vi "Configure Parameter to Measure.vi"(8 "error in (no error)":errorcluster, 10 "Sparameters (string)":string[](array[string]), 11 "VNA-PNA in":refnum<class "VNA-PNA.lvclass">) -> (0 "error out":errorcluster, 3 "VNA-PNA out":refnum<class "VNA-PNA.lvclass">)   [LabVIEW 2020, in "VNA-PNA.lvclass"]
doc: "Configures the active trace.\nIt creates the trace and sets the S paramert and mode."
uses:
  VNA-PNA.lvclass
  C:/Sandbox/RF Bench/Source Code/WiSpry Test Framework/Instruments/Vector Network Analyzer/Vector Network Analyzer.lvclass
  C:/Sandbox/RF Bench/Source Code/WiSpry Test Framework/Instruments/Instrument.lvclass
  Vector Network Analyzer.lvclass/Vector Network Analyzer.ctl
  Instrument.lvclass/Instrument.ctl
  Vector Network Analyzer.lvclass
  Instrument.lvclass
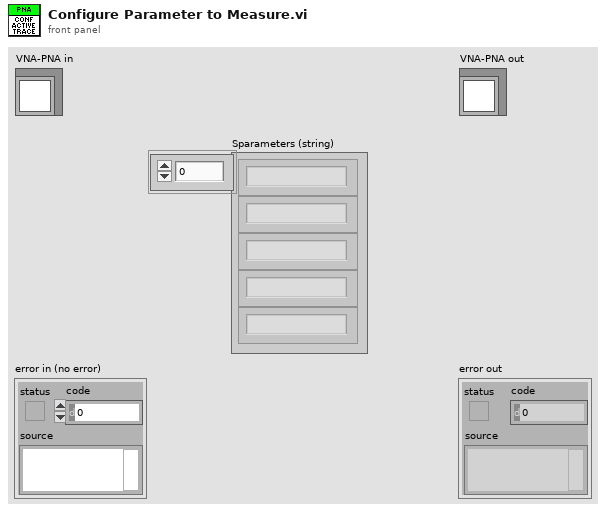
[diagram p1: front panel]
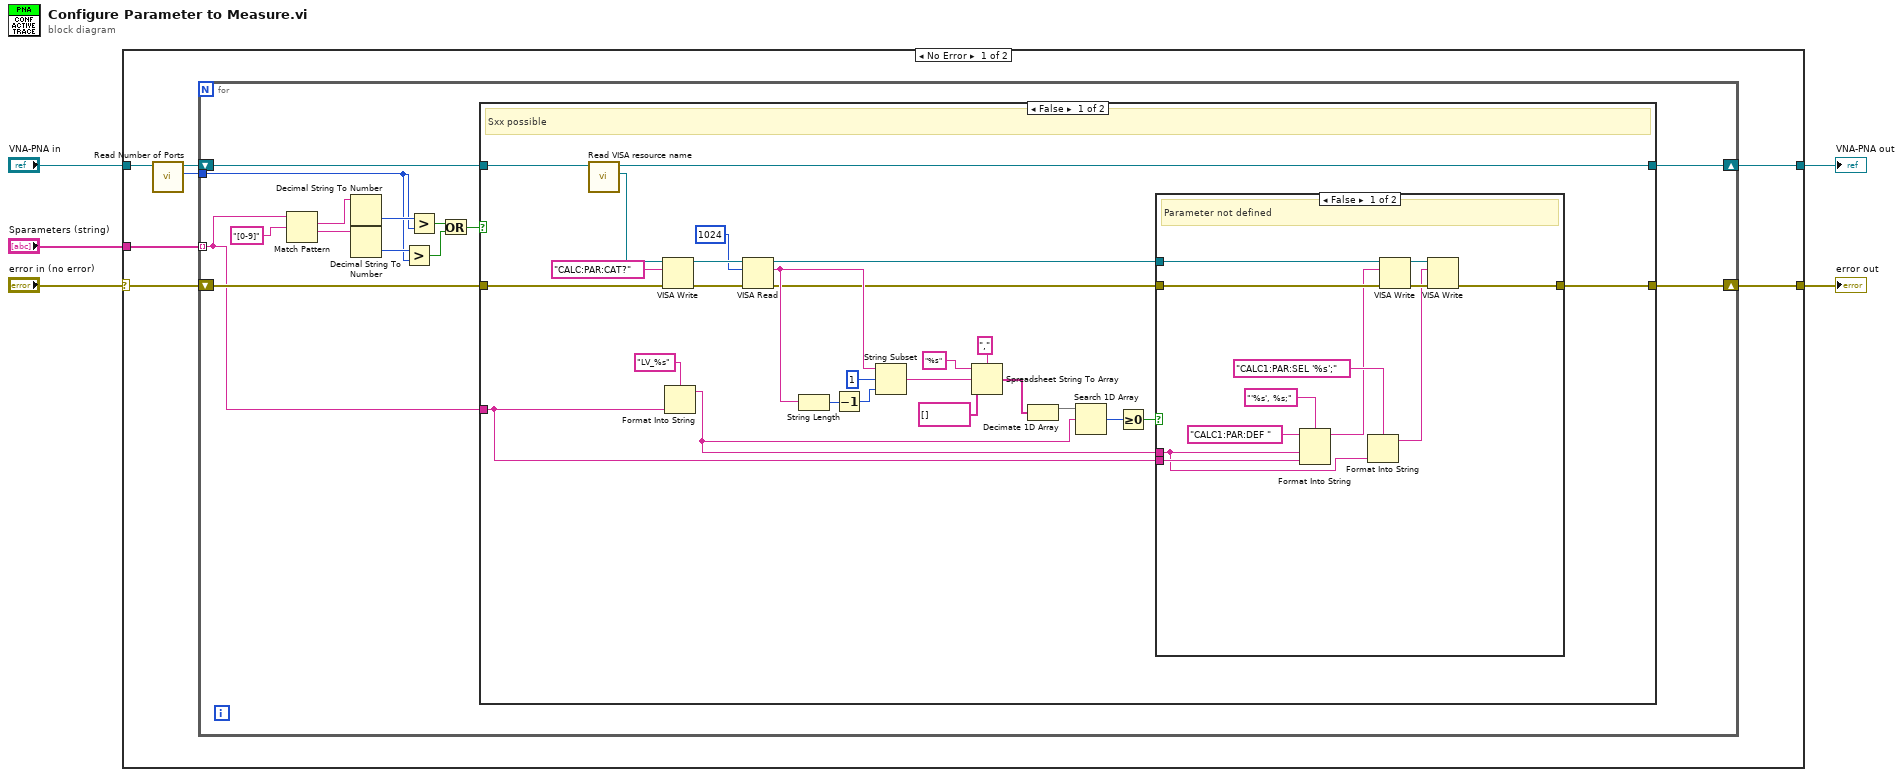
[diagram p0: block diagram]
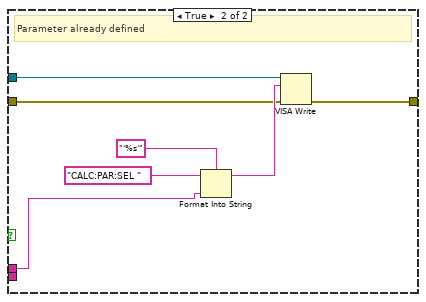
[diagram p2: hidden frame]
diagram:
  n1 = case shown="No Error" "error in (no error)" {
    selector: "error in (no error)" -> [w9 w75]
    tunnel: "VNA-PNA in" -> [w12 w74]
    tunnel: [w8 w75] -> w3
    tunnel: [w7 w74] -> w2
    tunnel: "Sparameters (string)" -> [w6 _]
    frame No Error {
      n2 = call "Read Number of Ports.vi"("Vector Network Analyzer in"=w12) -> ("Number of Ports"=w11:i32, "Vector Network Analyzer out"=w10:refnum<class "VNA-PNA.lvclass">)  [unwired: 9 in]
      n3 = for {
        tunnel: w11 -> [w21]
        shift-right: [w14] -> w7
        shift-left: w10 -> [w17]
        shift-right: [w15] -> w8
        shift-left: w9 -> [w16]
        tunnel: w6 -> [w13] mode=indexing
        n4 = Match Pattern(string=w13, regular expression="[0-9]") -> (match substring=w25:string, after substring=w24:string)  [unwired: 1 in, 2 out]
        n5 = Decimal String To Number(string=w25) -> (number=w23:i32)  [unwired: 2 in, 1 out]
        n6 = Decimal String To Number(string=w24) -> (number=w22:i32)  [unwired: 2 in, 1 out]
        n7 = Greater?(x=w22, y=w21) -> (0:w19:bool)
        n8 = Greater?(x=w23, y=w21) -> (0:w20:bool)
        n9 = Or(x=w20, y=w19) -> (x .or. y?=w18:bool)
        n10 = case shown="False" w18 {
          tunnel: w17 -> [w51 w73]
          tunnel: w16 -> [w46 w72]
          tunnel: w13 -> [w48 _]
          tunnel: [w49 w72] -> w15
          tunnel: [w50 w73] -> w14
          frame False {
            # "Sxx possible"
            n11 = call "Read VISA resource name.vi"("Instrument in"=w51) -> ("VISA resource name"=w47:refnum<visa-resource-name>, "Instrument out"=w50:refnum<class "VNA-PNA.lvclass">)  [unwired: 9 in]
            n12 = VISA Write(VISA resource name=w47, write buffer="CALC:PAR:CAT?", error in (no error)=w46) -> (VISA resource name out=w43:refnum<visa-resource-name>, error out=w44:errorcluster)  [unwired: 1 out]
            n13 = Format Into String(format string="LV_%s" ("initial string"), w48) -> (resulting string=w28:string)  [unwired: 2 in, 1 out]
            n14 = VISA Read(VISA resource name=w43, byte count=u32 1024, error in (no error)=w44) -> (VISA resource name out=w29:refnum<visa-resource-name>, read buffer=w38:string, error out=w31:errorcluster)  [unwired: 1 out]
            n15 = String Length(string=w38) -> (length=w39:i32)
            n16 = Decrement(x=w39) -> (x-1=w36:i32)
            n17 = String Subset(string=w38, offset (0)=1, length (rest)=w36) -> (substring=w35:string)
            n18 = Spreadsheet String To Array(delimiter (Tab)=",", format string="%s", spreadsheet string=w35, array type (2D Dbl)=string[] []) -> (array=w32:string[])
            n19 = Decimate 1D Array(w32) -> (w27:string[])  [unwired: 1 out]
            n20 = Search 1D Array(1D array=w27, element=w28) -> (index of element=w33:i32)  [unwired: 1 in]
            n21 = Greater Or Equal To 0?(x=w33) -> (x >= 0?=w30:bool)
            n22 = case shown="False" w30 {
              tunnel: [w53 w65] -> w49
              tunnel: w48 -> [w64 _]
              tunnel: w28 -> [w60 w68]
              tunnel: w31 -> [w59 w67]
              tunnel: w29 -> [w58 w66]
              frame False {
                # "Parameter not defined"
                n23 = Format Into String(format string="'%s', %s;", initial string="CALC1:PAR:DEF ", w60, w64) -> (resulting string=w57:string)  [unwired: 1 in, 1 out]
                n24 = Format Into String(format string="CALC1:PAR:SEL '%s';", w60) -> (resulting string=w54:string)  [unwired: 2 in, 1 out]
                n25 = VISA Write(VISA resource name=w58, write buffer=w57, error in (no error)=w59) -> (VISA resource name out=w55:refnum<visa-resource-name>, error out=w56:errorcluster)  [unwired: 1 out]
                n26 = VISA Write(VISA resource name=w55, write buffer=w54, error in (no error)=w56) -> (error out=w53:errorcluster)  [unwired: 2 out]
              }
              frame True {
                # "Parameter already defined"
                n27 = Format Into String(format string="'%s'", initial string="CALC:PAR:SEL ", w68) -> (resulting string=w69:string)  [unwired: 1 in, 1 out]
                n28 = VISA Write(VISA resource name=w66, write buffer=w69, error in (no error)=w67) -> (error out=w65:errorcluster)  [unwired: 2 out]
              }
            }
          }
          frame True {
            # "Add error handler"
            # "Sxx higher than ports"
          }
        }
      }
    }
    frame Error {
    }
  }
  "error out" <- w3
  "VNA-PNA out" <- w2
